vi "AndorAcqSingleImgToFile.vi"(6 "Image Name":string, 7 "Image Path":path, 8 "error in (no error)":errorcluster, 10 "Colormap":u16, 11 "Format":u16) -> (0 "error out":errorcluster)   [LabVIEW 2018, in "AndorOWN.lvlib"]
uses:
  AndorOWN.lvlib
  Andor SDK/AndorSDK.lvlib
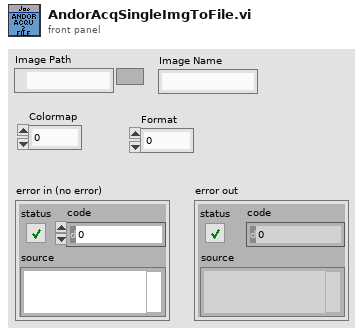
[diagram p1: front panel]
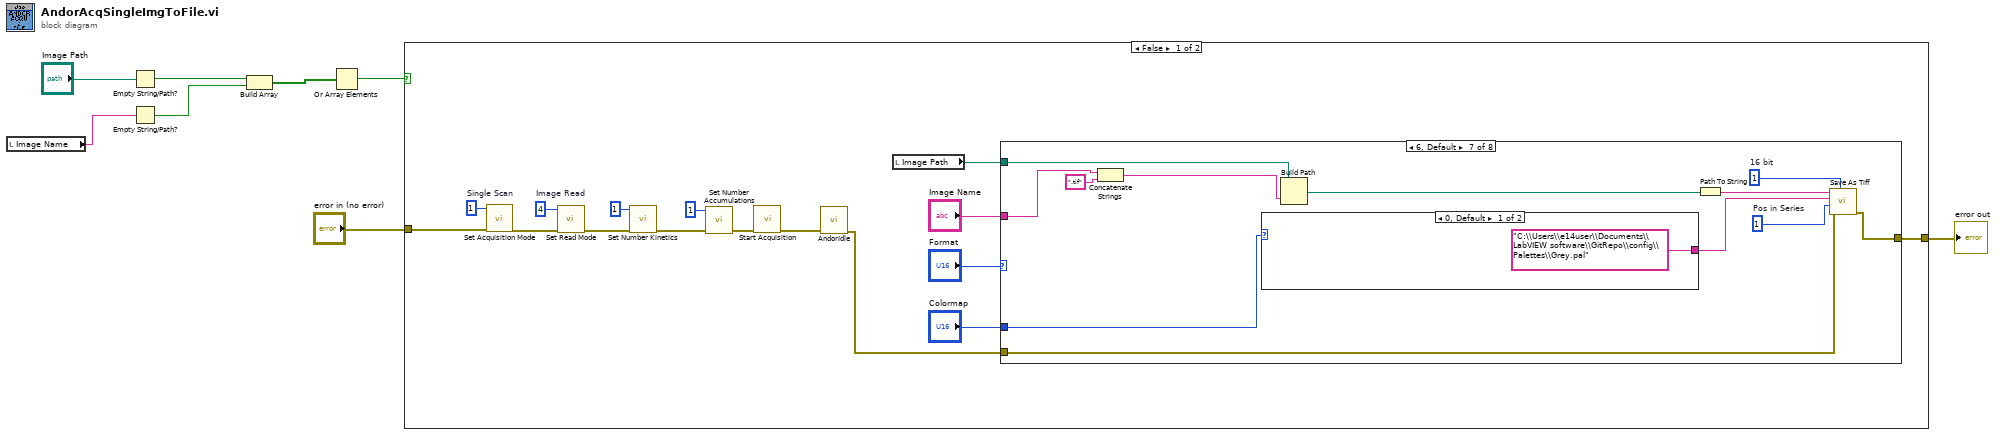
[diagram p0: block diagram]
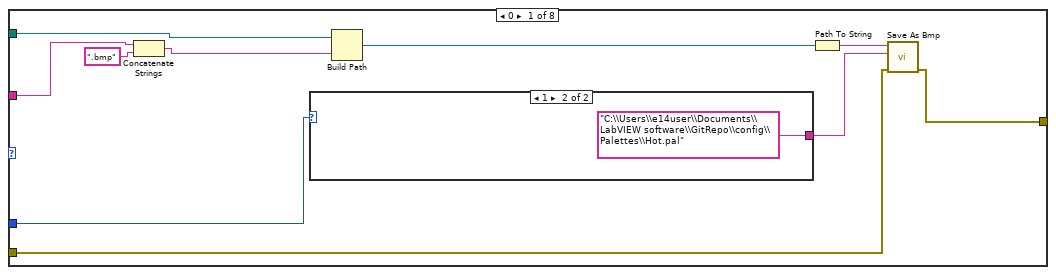
[diagram p2: hidden frame]
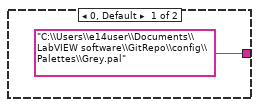
[diagram p3: hidden frame]
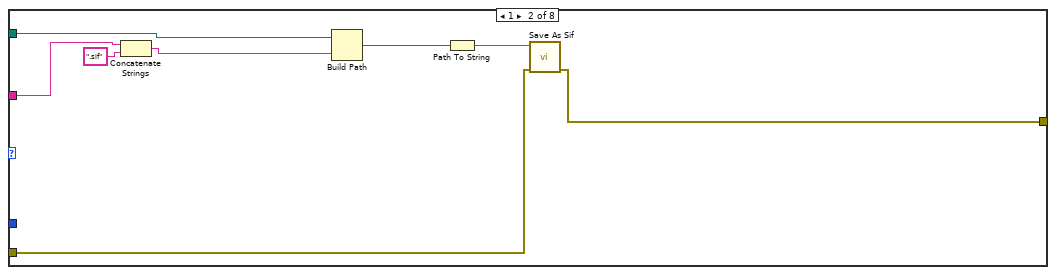
[diagram p4: hidden frame]
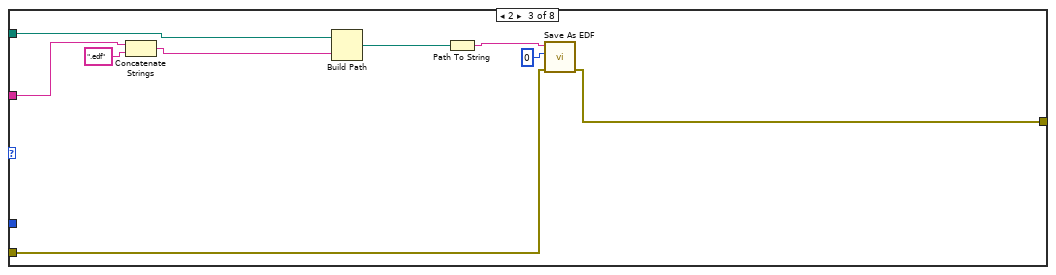
[diagram p5: hidden frame]
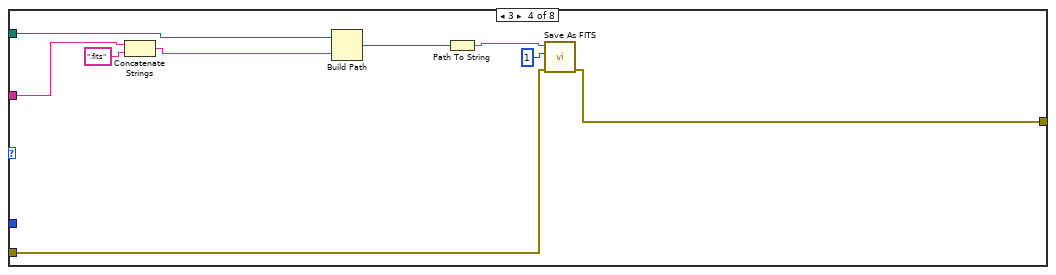
[diagram p6: hidden frame]
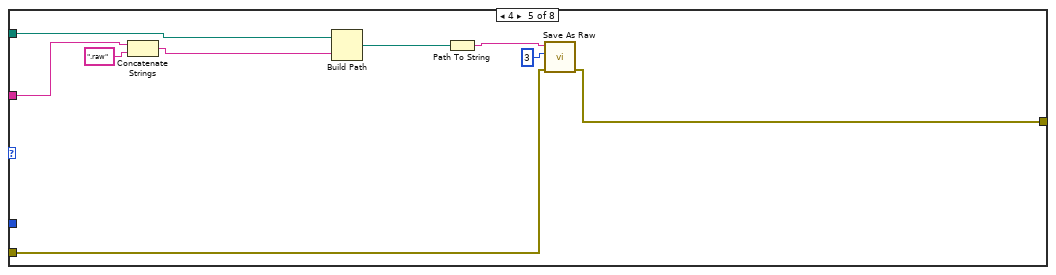
[diagram p7: hidden frame]
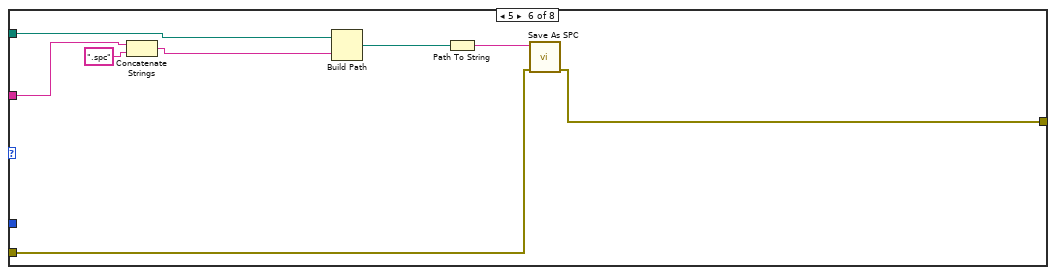
[diagram p8: hidden frame]
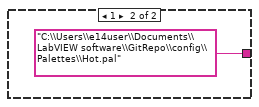
[diagram p9: hidden frame]
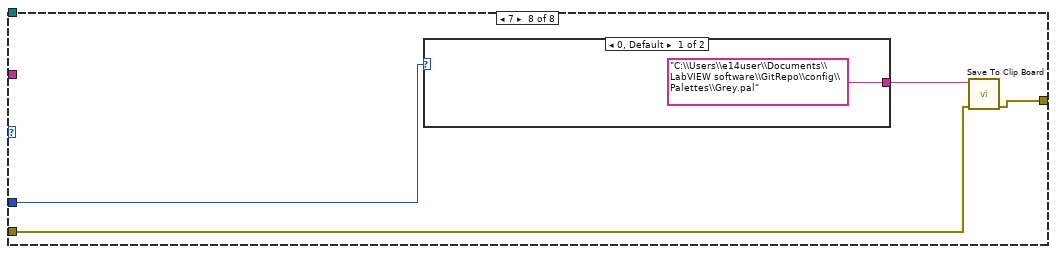
[diagram p10: hidden frame]
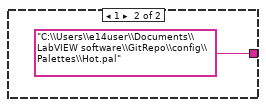
[diagram p11: hidden frame]
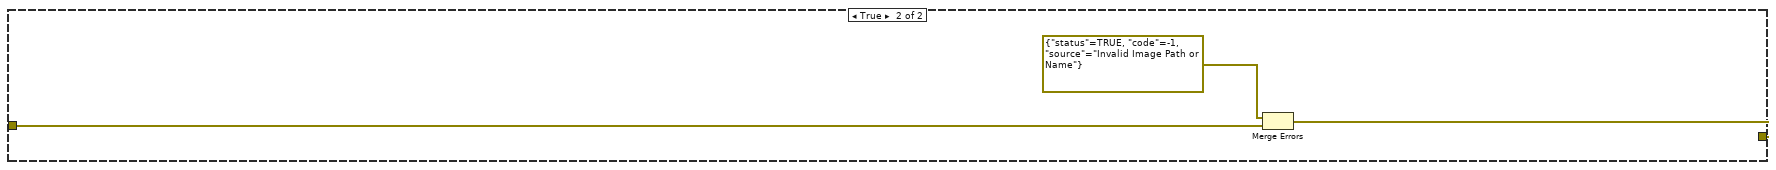
[diagram p12: hidden frame]
diagram:
  n1 = local read "Image Name"() -> (w3:string)
  n2 = Empty String/Path?(string/path="Image Path") -> (empty?=w5:bool)
  n3 = Empty String/Path?(string/path=w3) -> (empty?=w4:bool)
  n4 = Build Array(w5, w4) -> (w7:bool[])
  n5 = Or Array Elements(Boolean array=w7) -> (logical OR=w8:bool)
  n6 = case shown="False" w8 {
    tunnel: "error in (no error)" -> [w21 w102]
    tunnel: [w9 w101] -> w1
    frame False {
      w19 = 4  # Image Read
      w20 = 1  # Single Scan
      n7 = call "Set Acquisition Mode.vi"("error in (no error)"=w21, "mode"=w20) -> ("error out"=w22:errorcluster)  [unwired: 8 in, 1 out]
      n8 = call "Set Read Mode.vi"("error in (no error)"=w22, "mode"=w19) -> ("error out"=w23:errorcluster)  [unwired: 8 in, 1 out]
      n9 = call "Set Number Kinetics.vi"("error in (no error)"=w23, "number"=1) -> ("error out"=w24:errorcluster)  [unwired: 8 in, 1 out]
      n10 = call "Set Number Accumulations.vi"("error in (no error)"=w24, "number"=1) -> ("error out"=w12:errorcluster)  [unwired: 8 in, 1 out]
      n11 = call "Start Acquisition.vi"("error in (no error)"=w12) -> ("error out"=w11:errorcluster)  [unwired: 9 in, 1 out]
      n12 = call "AndorIdle.vi"("error in (no error)"=w11) -> ("error out"=w10:errorcluster)  [unwired: 9 in, 1 out]
      n13 = local read "Image Path"() -> (w13:path)
      n14 = case shown="6, Default" "Format" {
        tunnel: w13 -> [w34 w44 w53 w62 w71 w79 w91 _]
        tunnel: "Image Name" -> [w33 w43 w52 w61 w70 w78 w90 _]
        tunnel: "Colormap" -> [w27 _ _ _ _ _ w82 w96]
        tunnel: w10 -> [w26 w38 w46 w55 w64 w73 w81 w94]
        tunnel: [w25 w37 w45 w54 w63 w72 w80 w95] -> w9
        frame 0 {
          n15 = Concatenate Strings(w33, ".bmp" ("string")) -> (w31:string)
          n16 = case shown="1" w27 {
            tunnel: ["C:\\Users\\e14user\\Documents\\LabVIEW software\\GitRepo\\config\\Palettes\\Grey.pal" "C:\\Users\\e14user\\Documents\\LabVIEW software\\GitRepo\\config\\Palettes\\Hot.pal"] -> w28
            frame 0, Default {
            }
            frame 1 {
            }
          }
          n17 = Build Path(base path=w34, name or relative path=w31) -> (appended path=w30:path)
          n18 = Path To String(path=w30) -> (string=w29:string)
          n19 = call "Save As Bmp.vi"("error in (no error)"=w26, "palette"=w28, "path"=w29) -> ("error out"=w25:errorcluster)  [unwired: 5 in, 3 out]
        }
        frame 1 {
          n20 = Concatenate Strings(w43, ".sif" ("string")) -> (w41:string)
          n21 = Build Path(base path=w44, name or relative path=w41) -> (appended path=w39:path)
          n22 = Path To String(path=w39) -> (string=w40:string)
          n23 = call "Save As Sif.vi"("error in (no error)"=w38, "path"=w40) -> ("error out"=w37:errorcluster)  [unwired: 7 in, 2 out]
        }
        frame 2 {
          n24 = Concatenate Strings(w52, ".edf" ("string")) -> (w50:string)
          n25 = Build Path(base path=w53, name or relative path=w50) -> (appended path=w49:path)
          n26 = Path To String(path=w49) -> (string=w48:string)
          n27 = call "Save As EDF.vi"("error in (no error)"=w46, "iMode"=0, "szPath"=w48) -> ("error out"=w45:errorcluster)  [unwired: 6 in, 2 out]
        }
        frame 3 {
          n28 = Concatenate Strings(w61, ".fits" ("string")) -> (w59:string)
          n29 = Build Path(base path=w62, name or relative path=w59) -> (appended path=w58:path)
          n30 = Path To String(path=w58) -> (string=w57:string)
          n31 = call "Save As FITS.vi"("error in (no error)"=w55, "typ"=1, "szFileTitle"=w57) -> ("error out"=w54:errorcluster)  [unwired: 6 in, 2 out]
        }
        frame 4 {
          n32 = Concatenate Strings(w70, ".raw" ("string")) -> (w68:string)
          n33 = Build Path(base path=w71, name or relative path=w68) -> (appended path=w67:path)
          n34 = Path To String(path=w67) -> (string=w66:string)
          n35 = call "Save As Raw.vi"("error in (no error)"=w64, "typ"=3, "szFileTitle"=w66) -> ("error out"=w63:errorcluster)  [unwired: 6 in, 2 out]
        }
        frame 5 {
          n36 = Concatenate Strings(w78, ".spc" ("string")) -> (w76:string)
          n37 = Build Path(base path=w79, name or relative path=w76) -> (appended path=w75:path)
          n38 = Path To String(path=w75) -> (string=w74:string)
          n39 = call "Save As SPC.vi"("error in (no error)"=w73, "path"=w74) -> ("error out"=w72:errorcluster)  [unwired: 7 in, 2 out]
        }
        frame 6, Default {
          w83 = 1  # 16 bit
          w86 = 1  # Pos in Series
          n40 = Concatenate Strings(w90, ".tif" ("string")) -> (w88:string)
          n41 = case shown="0, Default" w82 {
            tunnel: ["C:\\Users\\e14user\\Documents\\LabVIEW software\\GitRepo\\config\\Palettes\\Grey.pal" "C:\\Users\\e14user\\Documents\\LabVIEW software\\GitRepo\\config\\Palettes\\Hot.pal"] -> w84
            frame 0, Default {
            }
            frame 1 {
            }
          }
          n42 = Build Path(base path=w91, name or relative path=w88) -> (appended path=w87:path)
          n43 = Path To String(path=w87) -> (string=w85:string)
          n44 = call "Save As Tiff.vi"("typ"=w83, "error in (no error)"=w81, "position"=w86, "palette"=w84, "path"=w85) -> ("error out"=w80:errorcluster)  [unwired: 3 in, 3 out]
        }
        frame 7 {
          n45 = case shown="0, Default" w96 {
            tunnel: ["C:\\Users\\e14user\\Documents\\LabVIEW software\\GitRepo\\config\\Palettes\\Grey.pal" "C:\\Users\\e14user\\Documents\\LabVIEW software\\GitRepo\\config\\Palettes\\Hot.pal"] -> w97
            frame 0, Default {
            }
            frame 1 {
            }
          }
          n46 = call "Save To Clip Board.vi"("error in (no error)"=w94, "palette"=w97) -> ("error out"=w95:errorcluster)  [unwired: 7 in, 2 out]
        }
      }
    }
    frame True {
      n47 = Merge Errors(errorcluster {"status"=TRUE, "code"=-1, "source"="Invalid Image Path or Name"} ("error constant"), w102) -> (w101:errorcluster)
    }
  }
  "error out" <- w1
